vi "CreateCommunication.vi"(8 "error in (no error)":errorcluster) -> (0 "error out":errorcluster, 3 "Message Queues out":T1)   [LabVIEW 2017, in "Server.lvlib" / "Message Queue.lvlib"]
doc: "Creates all Queues and User Events and stores them in References Cluster."
uses:
  Message Queue.lvlib
  CommReferences.ctl
  MessageCluster.ctl
  EnqueueMessage(Single).vi
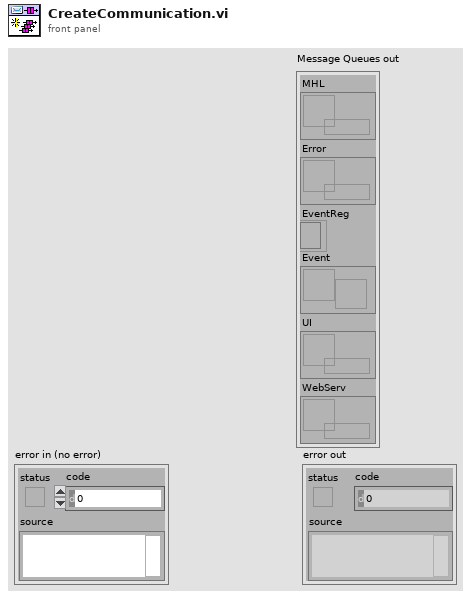
[diagram p1: front panel]
types:
  T1 = typedef "Server.lvlib/Message Queue.lvlib/CommReferences.ctl" = cluster{"MHL":refnum<queue>, "Error":refnum<queue>, "EventReg":refnum<event-registration>, "Event":refnum<user-event>, "UI":refnum<queue>, "WebServ":refnum<queue>}
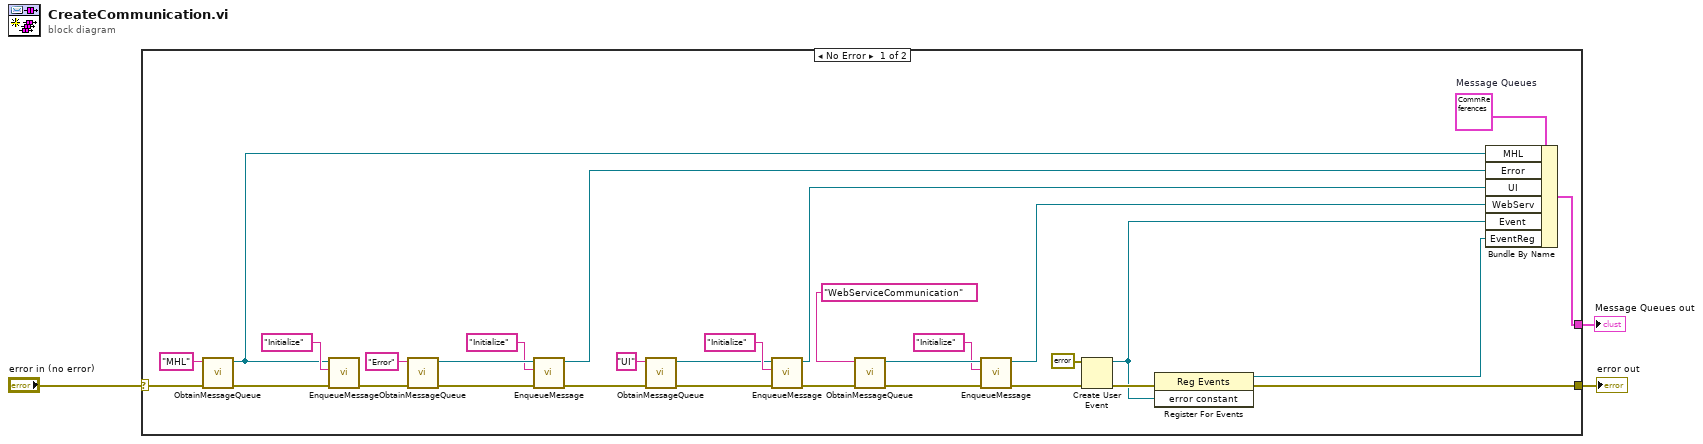
[diagram p0: block diagram]
diagram:
  n1 = case shown="No Error" "error in (no error)" {
    selector: "error in (no error)" -> [w32 w35]
    tunnel: [w20 w35] -> w3
    tunnel: [w33 _] -> w2
    frame No Error {
      w34 = T1 {"MHL"=refnum, "Error"=refnum, "EventReg"=refnum, "Event"=refnum, "UI"=refnum, "WebServ"=refnum}  # Message Queues
      n2 = call "ObtainMessageQueue.vi"("error in (no error)"=w32, "Name"="MHL") -> ("error out"=w31:errorcluster, "Message Queue"=w29:refnum<queue>)  [unwired: 8 in]
      n3 = call-poly "EnqueueMessage.vi"("error in (no error)"=w31, "Message"="Initialize", "Message Queue"=w29) -> ("error out"=w4:errorcluster)  [unwired: 7 in, 1 out]
      n4 = call "ObtainMessageQueue.vi"("error in (no error)"=w4, "Name"="Error") -> ("error out"=w25:errorcluster, "Message Queue"=w26:refnum<queue>)  [unwired: 8 in]
      n5 = call-poly "EnqueueMessage.vi"("error in (no error)"=w25, "Message"="Initialize", "Message Queue"=w26) -> ("error out"=w15:errorcluster, "dup Message Queue"=w23:refnum<queue>)  [unwired: 7 in]
      n6 = call "ObtainMessageQueue.vi"("error in (no error)"=w15, "Name"="UI") -> ("error out"=w18:errorcluster, "Message Queue"=w17:refnum<queue>)  [unwired: 8 in]
      n7 = call-poly "EnqueueMessage.vi"("error in (no error)"=w18, "Message"="Initialize", "Message Queue"=w17) -> ("error out"=w9:errorcluster, "dup Message Queue"=w14:refnum<queue>)  [unwired: 7 in]
      n8 = call "ObtainMessageQueue.vi"("error in (no error)"=w9, "Name"="WebServiceCommunication") -> ("error out"=w11:errorcluster, "Message Queue"=w12:refnum<queue>)  [unwired: 8 in]
      n9 = call-poly "EnqueueMessage.vi"("error in (no error)"=w11, "Message"="Initialize", "Message Queue"=w12) -> ("error out"=w8:errorcluster, "dup Message Queue"=w5:refnum<queue>)  [unwired: 7 in]
      n10 = Create User Event(user event datatype=errorcluster {"status"=FALSE, "code"=0, "source"=""} ("error constant"), error in=w8) -> (user event=w6:refnum<user-event>, error out=w22:errorcluster)
      n11 = register-events(error in=w22, w6) -> (reference out=w7:refnum<event-registration>, error out=w20:errorcluster)  [unwired: 1 in]
      n12 = Bundle By Name(cluster=w34, "MHL"=w29, "Error"=w23, "UI"=w14, "WebServ"=w5, "Event"=w6, "EventReg"=w7) -> (w33:T1)
    }
    frame Error {
    }
  }
  "Message Queues out" <- w2
  "error out" <- w3
